vi "GlueMovePickPlace.vi"() -> ()   [LabVIEW 2019]
panel:
  in  "PatternAngleInDeg":dbl=90.0 format="%#_13g"
  out "Status":string
  in  "stop":bool
  in  "Start with Sequence":bool
  in  "Glue":bool
  out "Comm":string
  out "Speed":dbl format="%#_13g"
  out "Time(ms)":dbl
  in  "OriginZ":dbl=71.78 format="%#_13g"
  in  "OriginY":dbl=804.07 format="%#_13g"
  in  "OriginX":dbl=127.553 format="%#_13g"
  in  "Pressure":dbl[](array[numeric])=[27.0, 27.0, 27.0, 27.0]
  in  "Path":path=path "C:/Users/TTUHEP/Documents/LabVIEW/Data/Patterns/PCB_base_Dec21_Combined.ngc"
  in  "Serial Configuration":T1={"Baud Rate "=115200, "Parity "=0, "Data Bits "=8, "Stop Bits"=10} {"Stop Bits" items=["1.0"=10, "1.5"=15, "2.0"=20]; "Data Bits" items=["7"=7, "8"=8]; "Parity" items=["None", "Odd", "Even"]; "Baud Rate" items=["9600"=9600, "19200"=19200, "38400"=38400, "115200"=115200]}
  in  "VISA resource name":refnum<visa-resource-name>="COM6"
  in  "GoToZero":bool=TRUE
  in  "MoveToToolDropPosition":bool=TRUE
  in  "DropTool":bool=TRUE
  in  "DropPlate":bool=TRUE
  in  "MoveToAssemblyPosition":bool=TRUE
  in  "PickPlate":bool=TRUE
  in  "MoveToPlatePosition":bool=TRUE
  in  "PickTool":bool=TRUE
  in  "MoveToToolPosition":bool=TRUE
  out "Final":string
  in  "Move Z first 5":bool=TRUE
  in  "Absolute 5":bool=TRUE
  in  "SpeedZ (mm/s) 5":dbl=10.0
  in  "SpeedXY (mm/s) 5":dbl=100.0
  in  "Z 5":dbl
  in  "Y 5":dbl
  in  "X 5":dbl
  out "sensor on? 4":bool
  out "Tool Position drop":string
  in  "Move Z first 4":bool
  in  "Absolute 4":bool=TRUE
  in  "SpeedZ (mm/s) 4":dbl=10.0
  in  "SpeedXY (mm/s) 4":dbl=100.0
  in  "Z 4":dbl
  in  "Y 4":dbl=885.01
  in  "X 4":dbl=956.907
  out "sensor on? 3":bool
  out "Assembly Position":string
  in  "Move Z first 3":bool
  in  "Absolute 3":bool=TRUE
  in  "SpeedZ (mm/s) 3":dbl=10.0
  in  "SpeedXY (mm/s) 3":dbl=100.0
  in  "Z 3":dbl
  in  "Y 3":dbl=975.071
  in  "X 3":dbl=553.52
  out "sensor on? 2":bool
  out "sensor on?":bool
  out "error out":errorcluster
  out "Plate Position":string
  in  "Move Z first 2":bool
  in  "Absolute 2":bool=TRUE
  in  "SpeedZ (mm/s) 2":dbl=10.0
  in  "SpeedXY (mm/s) 2":dbl=100.0
  in  "Z 2":dbl
  in  "Y 2":dbl=978.581
  in  "X 2":dbl=779.31
  out "Tool Position":string
  in  "Move Z first":bool
  in  "Absolute":bool=TRUE
  in  "SpeedZ (mm/s)":dbl=10.0
  in  "SpeedXY (mm/s)":dbl=100.0
  in  "Z":dbl
  in  "Y":dbl=885.01
  in  "X":dbl=956.907
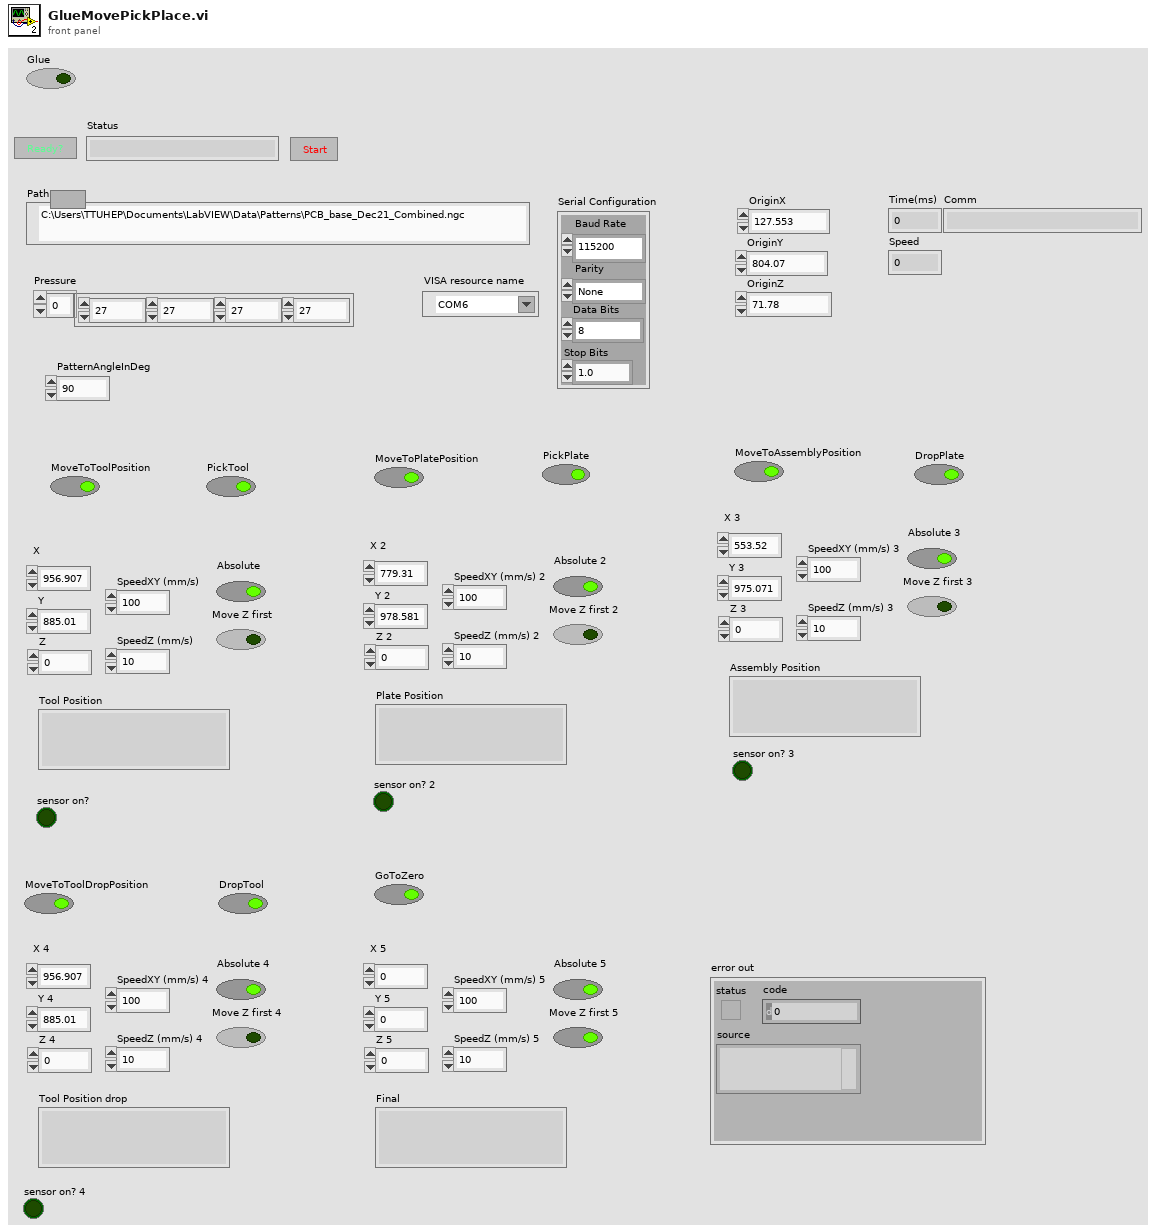
[diagram p1: front panel]
types:
  T1 = cluster{"Baud Rate ":u32, "Parity ":u16, "Data Bits ":u16, "Stop Bits":u16}
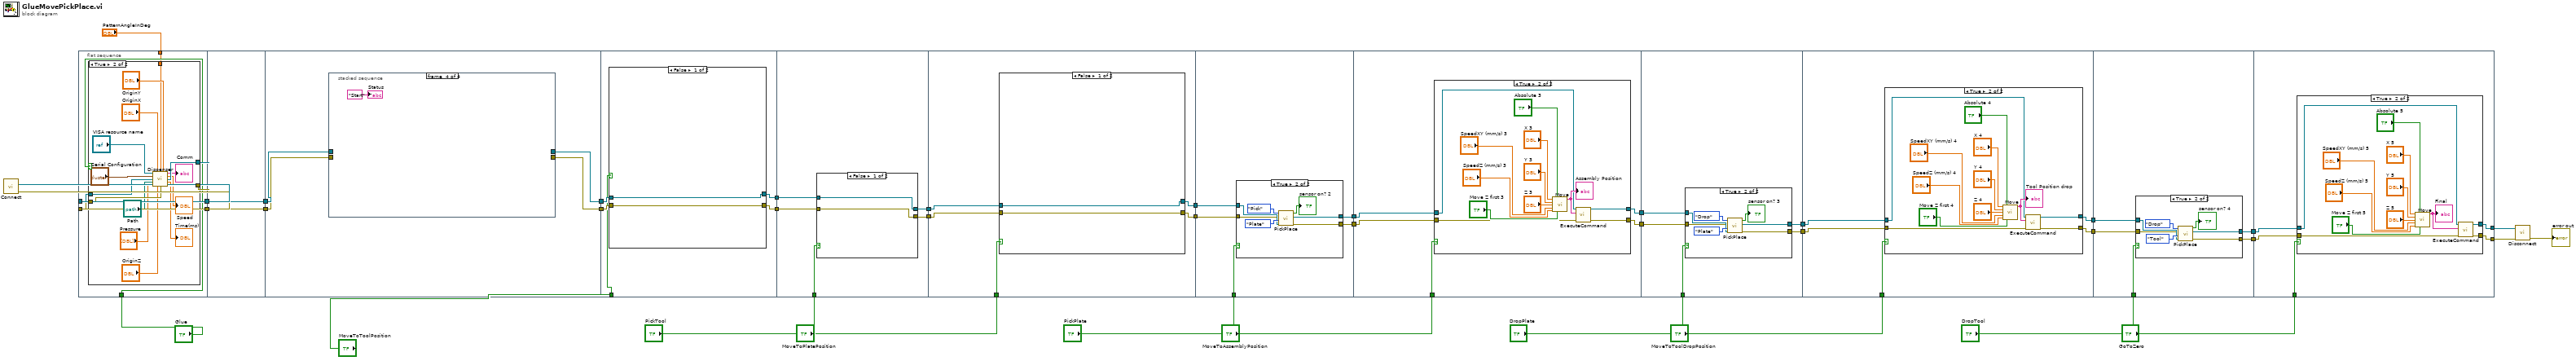
[diagram p0: block diagram]
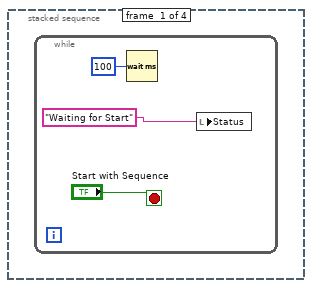
[diagram p3: hidden frame]
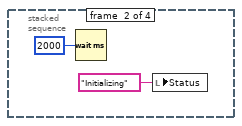
[diagram p4: hidden frame]
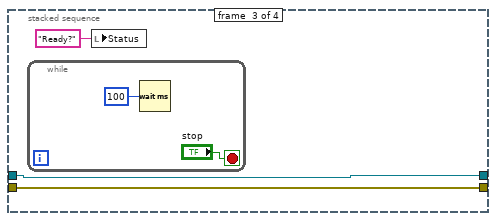
[diagram p5: hidden frame]
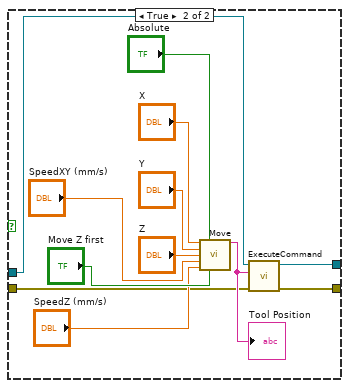
[diagram p6: hidden frame]
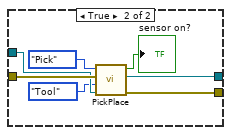
[diagram p7: hidden frame]
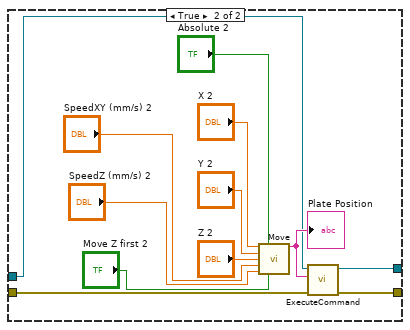
[diagram p8: hidden frame]
diagram:
  n1 = call "Connect.vi"() -> ("error out"=w36:errorcluster, "controller"=w37:refnum<k24>)  [unwired: 10 in]
  n2 = flat-sequence {
    tunnel: w36 -> [w41]
    tunnel: w37 -> [w44]
    tunnel: [w43] -> w5
    tunnel: [w42] -> w3
    tunnel: "Glue" -> [w40]
    tunnel: "PatternAngleInDeg" -> [w39]
    tunnel: w5 -> [w62]
    tunnel: [w62] -> w4
    tunnel: w3 -> [w63]
    tunnel: [w63] -> w2
    tunnel: w4 -> [w67]
    tunnel: [w66] -> w7
    tunnel: w2 -> [w65]
    tunnel: [w64] -> w6
    tunnel: [w81] -> w33
    tunnel: [w80] -> w31
    tunnel: "MoveToToolPosition" -> [w79]
    tunnel: w7 -> [w83]
    tunnel: w6 -> [w82]
    tunnel: w33 -> [w102]
    tunnel: [w99] -> w32
    tunnel: w31 -> [w101]
    tunnel: [w100] -> w30
    tunnel: "PickTool" -> [w98]
    tunnel: w32 -> [w115]
    tunnel: w30 -> [w116]
    tunnel: [w114] -> w29
    tunnel: [w113] -> w28
    tunnel: "MoveToPlatePosition" -> [w112]
    tunnel: w29 -> [w134]
    tunnel: w28 -> [w135]
    tunnel: [w132] -> w27
    tunnel: [w133] -> w26
    tunnel: "PickPlate" -> [w131]
    tunnel: w27 -> [w148]
    tunnel: w26 -> [w149]
    tunnel: [w147] -> w25
    tunnel: [w146] -> w24
    tunnel: "MoveToAssemblyPosition" -> [w145]
    tunnel: w25 -> [w165]
    tunnel: w24 -> [w167]
    tunnel: [w166] -> w23
    tunnel: [w168] -> w22
    tunnel: "DropPlate" -> [w164]
    tunnel: w23 -> [w181]
    tunnel: w22 -> [w182]
    tunnel: [w179] -> w21
    tunnel: [w180] -> w20
    tunnel: "MoveToToolDropPosition" -> [w178]
    tunnel: w21 -> [w200]
    tunnel: w20 -> [w201]
    tunnel: [w199] -> w19
    tunnel: [w198] -> w18
    tunnel: "DropTool" -> [w197]
    tunnel: [w213] -> w34
    tunnel: [w212] -> w35
    tunnel: w19 -> [w214]
    tunnel: w18 -> [w215]
    tunnel: "GoToZero" -> [w211]
    frame #0 {
      n3 = case shown="True" w40 {
        tunnel: w44 -> [w46 w61]
        tunnel: [w46 w60] -> w43
        tunnel: [w45 w59] -> w42
        tunnel: w41 -> [w45 w58]
        tunnel: w39 -> [_ w47]
        frame False {
        }
        frame True {
          n4 = call "Dispenser.vi"("VISA resource name"="VISA resource name", "X"="OriginX", "AngleInDeg"=w47, "Y"="OriginY", "Serial Configuration"="Serial Configuration", "controller in"=w61, "Path"="Path", "Pressure"="Pressure", "Z"="OriginZ", "error in (no error)"=w58) -> ("Comm"=→"Comm":string, "Speed"=→"Speed":dbl, "controller out"=w60:refnum<k24>, "Time(ms)"=→"Time(ms)":dbl, "error out"=w59:errorcluster)  [unwired: 1 in]
        }
      }
    }
    frame #1 {
    }
    frame #2 {
      n5 = stacked-sequence {
        tunnel: w67 -> [_ _ w74 _]
        tunnel: [_ _ w74 _] -> w66
        tunnel: w65 -> [_ _ w73 _]
        tunnel: [_ _ w73 _] -> w64
        frame #0 {
          n6 = while {
            stop <- "Start with Sequence" stop-if-true
            n7 = Wait (ms)(milliseconds to wait=u32 100) -> ()  [unwired: 1 out]
            n8 = local write "Status"("Waiting for Start") -> ()
          }
        }
        frame #1 {
          n9 = Wait (ms)(milliseconds to wait=u32 2000) -> ()  [unwired: 1 out]
          n10 = local write "Status"("Initializing" ("Status")) -> ()
        }
        frame #2 {
          n11 = while {
            stop <- "stop" stop-if-true
            n12 = Wait (ms)(milliseconds to wait=u32 100) -> ()  [unwired: 1 out]
          }
          n13 = local write "Status"("Ready?" ("Status")) -> ()
        }
        frame #3 {
          "Status" <- "Start" ("Status")
        }
      }
    }
    frame #3 {
      n14 = case shown="False" w79 {
        tunnel: w83 -> [w85 w89]
        tunnel: w82 -> [w84 w88]
        tunnel: [w84 w87] -> w81
        tunnel: [w85 w86] -> w80
        frame False {
        }
        frame True {
          n15 = call "Move.vi"("X"="X", "Absolute"="Absolute", "Y"="Y", "Z"="Z", "SpeedXY (mm/s)"="SpeedXY (mm/s)", "SpeedZ (mm/s)"="SpeedZ (mm/s)", "Move Z first"="Move Z first") -> ("Position Gcode"=w90:string)  [unwired: 8 in]
          "Tool Position" <- w90
          n16 = call "ExecuteCommand.vi"("error in (no error)"=w88, "Command Code"=w90, "controller in"=w89) -> ("error out"=w87:errorcluster, "controller out"=w86:refnum<k24>)  [unwired: 6 in, 1 out]
        }
      }
    }
    frame #4 {
      n17 = case shown="False" w98 {
        tunnel: w102 -> [w104 w110]
        tunnel: w101 -> [w103 w109]
        tunnel: [w103 w106] -> w100
        tunnel: [w104 w105] -> w99
        frame False {
        }
        frame True {
          n18 = call "PickPlace.vi"("controller"=w109, "Tool or Plate"=enum16{"Tool", "Plate"}."Tool", "error in (no error)"=w110, "Pick or Drop"=enum16{"Pick", "Drop"}."Pick") -> ("error out"=w105:errorcluster, "controller out"=w106:refnum<k24>, "sensor on?"=→"sensor on?":bool)  [unwired: 1 in]
        }
      }
    }
    frame #5 {
      n19 = case shown="False" w112 {
        tunnel: w116 -> [w117 w122]
        tunnel: w115 -> [w118 w121]
        tunnel: [w118 w120] -> w114
        tunnel: [w117 w119] -> w113
        frame False {
        }
        frame True {
          n20 = call "Move.vi"("X"="X 2", "Absolute"="Absolute 2", "Y"="Y 2", "Z"="Z 2", "SpeedXY (mm/s)"="SpeedXY (mm/s) 2", "SpeedZ (mm/s)"="SpeedZ (mm/s) 2", "Move Z first"="Move Z first 2") -> ("Position Gcode"=w123:string)  [unwired: 8 in]
          "Plate Position" <- w123
          n21 = call "ExecuteCommand.vi"("error in (no error)"=w121, "Command Code"=w123, "controller in"=w122) -> ("error out"=w120:errorcluster, "controller out"=w119:refnum<k24>)  [unwired: 6 in, 1 out]
        }
      }
    }
    frame #6 {
      n22 = case shown="True" w131 {
        tunnel: w135 -> [w136 w141]
        tunnel: w134 -> [w137 w140]
        tunnel: [w136 w139] -> w133
        tunnel: [w137 w138] -> w132
        frame False {
        }
        frame True {
          n23 = call "PickPlace.vi"("controller"=w141, "Tool or Plate"=enum16{"Tool", "Plate"}."Plate", "error in (no error)"=w140, "Pick or Drop"=enum16{"Pick", "Drop"}."Pick") -> ("error out"=w138:errorcluster, "controller out"=w139:refnum<k24>, "sensor on?"=→"sensor on? 2":bool)  [unwired: 1 in]
        }
      }
    }
    frame #7 {
      n24 = case shown="True" w145 {
        tunnel: w149 -> [w151 w155]
        tunnel: w148 -> [w150 w154]
        tunnel: [w150 w153] -> w147
        tunnel: [w151 w152] -> w146
        frame False {
        }
        frame True {
          n25 = call "Move.vi"("X"="X 3", "Absolute"="Absolute 3", "Y"="Y 3", "Z"="Z 3", "SpeedXY (mm/s)"="SpeedXY (mm/s) 3", "SpeedZ (mm/s)"="SpeedZ (mm/s) 3", "Move Z first"="Move Z first 3") -> ("Position Gcode"=w156:string)  [unwired: 8 in]
          "Assembly Position" <- w156
          n26 = call "ExecuteCommand.vi"("error in (no error)"=w154, "Command Code"=w156, "controller in"=w155) -> ("error out"=w153:errorcluster, "controller out"=w152:refnum<k24>)  [unwired: 6 in, 1 out]
        }
      }
    }
    frame #8 {
      n27 = case shown="True" w164 {
        tunnel: [w169 w174] -> w168
        tunnel: w167 -> [w169 w173]
        tunnel: [w170 w172] -> w166
        tunnel: w165 -> [w170 w171]
        frame False {
        }
        frame True {
          n28 = call "PickPlace.vi"("controller"=w173, "Tool or Plate"=enum16{"Tool", "Plate"}."Plate", "error in (no error)"=w171, "Pick or Drop"=enum16{"Pick", "Drop"}."Drop") -> ("error out"=w172:errorcluster, "controller out"=w174:refnum<k24>, "sensor on?"=→"sensor on? 3":bool)  [unwired: 1 in]
        }
      }
    }
    frame #9 {
      n29 = case shown="True" w178 {
        tunnel: w182 -> [w183 w188]
        tunnel: w181 -> [w184 w187]
        tunnel: [w183 w186] -> w180
        tunnel: [w184 w185] -> w179
        frame False {
        }
        frame True {
          n30 = call "Move.vi"("X"="X 4", "Absolute"="Absolute 4", "Y"="Y 4", "Z"="Z 4", "SpeedXY (mm/s)"="SpeedXY (mm/s) 4", "SpeedZ (mm/s)"="SpeedZ (mm/s) 4", "Move Z first"="Move Z first 4") -> ("Position Gcode"=w189:string)  [unwired: 8 in]
          "Tool Position drop" <- w189
          n31 = call "ExecuteCommand.vi"("error in (no error)"=w187, "Command Code"=w189, "controller in"=w188) -> ("error out"=w185:errorcluster, "controller out"=w186:refnum<k24>)  [unwired: 6 in, 1 out]
        }
      }
    }
    frame #10 {
      n32 = case shown="True" w197 {
        tunnel: w201 -> [w202 w207]
        tunnel: w200 -> [w203 w206]
        tunnel: [w203 w205] -> w199
        tunnel: [w202 w204] -> w198
        frame False {
        }
        frame True {
          n33 = call "PickPlace.vi"("controller"=w207, "Tool or Plate"=enum16{"Tool", "Plate"}."Tool", "error in (no error)"=w206, "Pick or Drop"=enum16{"Pick", "Drop"}."Drop") -> ("error out"=w205:errorcluster, "controller out"=w204:refnum<k24>, "sensor on?"=→"sensor on? 4":bool)  [unwired: 1 in]
        }
      }
    }
    frame #11 {
      n34 = case shown="True" w211 {
        tunnel: w215 -> [w216 w221]
        tunnel: w214 -> [w217 w220]
        tunnel: [w216 w219] -> w213
        tunnel: [w217 w218] -> w212
        frame False {
        }
        frame True {
          n35 = call "Move.vi"("X"="X 5", "Absolute"="Absolute 5", "Y"="Y 5", "Z"="Z 5", "SpeedXY (mm/s)"="SpeedXY (mm/s) 5", "SpeedZ (mm/s)"="SpeedZ (mm/s) 5", "Move Z first"="Move Z first 5") -> ("Position Gcode"=w222:string)  [unwired: 8 in]
          "Final" <- w222
          n36 = call "ExecuteCommand.vi"("error in (no error)"=w220, "Command Code"=w222, "controller in"=w221) -> ("error out"=w218:errorcluster, "controller out"=w219:refnum<k24>)  [unwired: 6 in, 1 out]
        }
      }
    }
  }
  n37 = call "Disconnect.vi"("error in (no error)"=w35, "controller"=w34) -> ("error out"=→"error out":errorcluster)  [unwired: 9 in]
